vi "PC_time_to_GPS_time.vi"(0 "current PC time":timestamp) -> (1 "current GPS time":timestamp, 2 "GPS date/time string":string)   [LabVIEW 8.6]
panel:
  out "All data from ini file":string
  out "ini path":path
  out "Time_difference":string
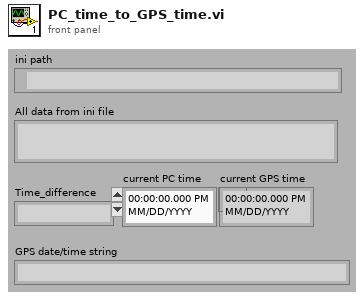
[diagram p1: front panel]
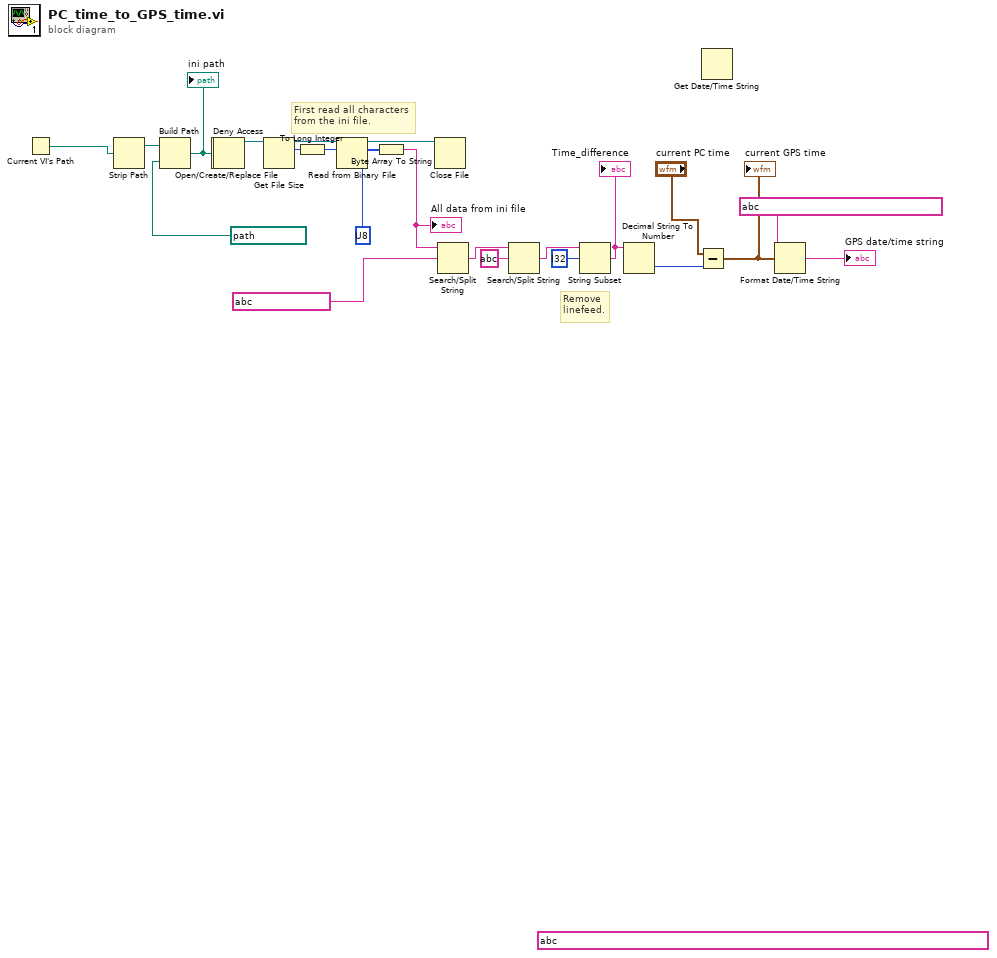
[diagram p0: block diagram]
diagram:
  (unwired) string ? ("format string")
  # "Remove\nlinefeed."
  # "First read all characters\nfrom the ini file."
  n1 = Current VI's Path() -> (path=w1:path)
  n2 = Strip Path(path=w1) -> (stripped path=w15:path)  [unwired: 1 out]
  n3 = Build Path(base path=w15, name or relative path=path ? ("configuration file path")) -> (appended path=w14:path)
  "ini path" <- w14
  n4 = Open/Create/Replace File(file path (use dialog)=w14) -> (refnum out=w17:refnum<file>, error out=w18:errorcluster)  [unwired: 5 in, 1 out]
  n5 = Deny Access(4:w18, 7:w17) -> (3:w24:refnum<file>)  [unwired: 1 in, 1 out]
  n6 = Get File Size(file=w24) -> (refnum out=w23:refnum<file>, size (in bytes)=w19:i64)  [unwired: 1 in, 1 out]
  n7 = To Long Integer(number=w19) -> (32bit integer=w22:i32)
  n8 = Read from Binary File(5:u8 ? ("byte stream type"), 10:w22, 11:w23) -> (2:w20:u8[], 3:w21:refnum<file>)  [unwired: 3 in, 2 out]
  n9 = Byte Array To String(unsigned byte array=w20) -> (string=w12:string)
  "All data from ini file" <- w12
  n10 = Close File(refnum=w21) -> ()  [unwired: 1 in, 2 out]
  n11 = Search/Split String(string=w12, search string/char (-)=string ?) -> (match + rest of string=w11:string)  [unwired: 1 in, 2 out]
  n12 = Search/Split String(string=w11, search string/char (-)=string ?) -> (match + rest of string=w8:string)  [unwired: 1 in, 2 out]
  n13 = String Subset(string=w8, offset (0)=i32 ?) -> (substring=w7:string)  [unwired: 1 in]
  "Time_difference" <- w7
  n14 = Decimal String To Number(string=w7) -> (number=w6:i32)  [unwired: 2 in, 1 out]
  n15 = Subtract(x="current PC time", y=w6) -> (x-y=w2:timestamp)
  "current GPS time" <- w2
  n16 = Get Date/Time String() -> ()  [unwired: 3 in, 2 out]
  n17 = Format Date/Time String(time format string (%c)=string ?, seconds (now)=w2) -> (date/time string=→"GPS date/time string":string)  [unwired: 1 out]
